vi "Change MFC Setpoints.vi"(8 "error in":errorcluster, 11 "Alicats":refnum<class "Alicat Device.lvclass">[](array[class])) -> (0 "error out":errorcluster)   [LabVIEW 2015]
uses:
  Devices/Alicat/Session Based/Alicat Device.lvclass
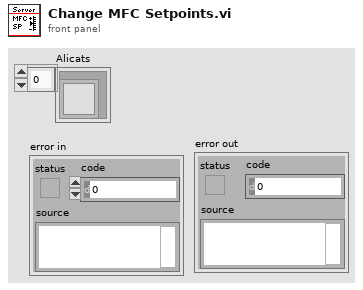
[diagram p1: front panel]
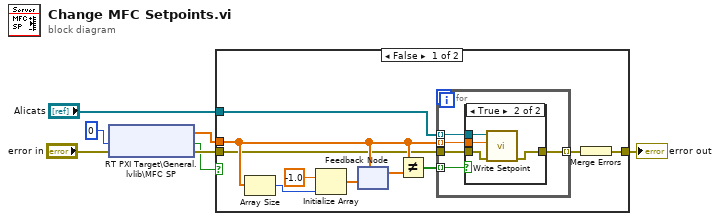
[diagram p0: block diagram]
diagram:
  n1 = shared-variable "RT PXI Target\\General.lvlib\\MFC SP"(error in="error in", 0 ("ms timeout (0)")) -> (w6:sgl[], error out=w5:errorcluster, w4:bool)
  n2 = case shown="False" w4 {
    tunnel: w5 -> [w11 w28]
    tunnel: w6 -> [w12 _]
    tunnel: [w9 w28] -> w3
    tunnel: "Alicats" -> [w8 _]
    frame False {
      n3 = Array Size(array=w12) -> (size(s)=w17:i32)
      n4 = Initialize Array(sgl -1.0 ("element"), w17) -> (w15:sgl[])
      n5 = feedback-in #1(w12) -> ()
      n6 = feedback #1(w15) -> (w14:sgl[])
      n7 = Not Equal?(x=w12, y=w14) -> (x != y?=w13:bool[])
      n8 = for {
        tunnel: w13 -> [w21] mode=indexing
        tunnel: w8 -> [w22] mode=indexing
        tunnel: w12 -> [w20] mode=indexing
        tunnel: w11 -> [w19]
        tunnel: [w18] -> w10 mode=indexing
        n9 = case shown="True" w21 {
          tunnel: w22 -> [_ w27]
          tunnel: w20 -> [_ w26]
          tunnel: w19 -> [w23 w24]
          tunnel: [w23 w25] -> w18
          frame False {
          }
          frame True {
            n10 = call "Write Setpoint.vi"("error in"=w24, "Setpoint"=w26, "Alicat Device in"=w27) -> ("error out"=w25:errorcluster)  [unwired: 6 in, 2 out]
          }
        }
      }
      n11 = Merge Errors(w10) -> (w9:errorcluster)
    }
    frame True {
    }
  }
  "error out" <- w3
